vi "Get Status Info [STS].vi"(7 "Micropulse # In":i32, 8 "error in (no error)":errorcluster, 10 "Request System Status":T1 caption="[STS]") -> (0 "error out":errorcluster, 5 "Micropulse # Out":i32)   [LabVIEW 2026, in "MicroPulse_Driver.lvlib"]
doc: "Request Parameters.\n\nFormat: STS <mode>\n\nDescription:\nFor backward compatibility STS -1 can be used to find out the information contained in a RST message without resetting the MicroPulse. Other modes can be used to request various parameters from the MicroPulse.\n\nParameters:\n<mode> : \n= 0 ¨ axis locations\n= 1 ¨ MPE settings\n= 2 ¨ BKL settings\n= 5 ¨ SPA settings\n= 6 ¨ Read status of input and output lines\n= 7 ¨ Time in seconds since last power-on, RST and SRST\n= 8 ¨ System information (see section 4.5)\n= 20 ¨ System temperature readings\n= 21 ¨ Output system log (see section 4.5)\n= 22 ¨ Erase system log (see section 4.5)\n= -1 ¨ RST message\n= -2 ¨ Copy of primary system RST message when in primary/secondary mode\n= -3 ¨ Copy of secondary system RST message when in primary/secondary mode\n\nReply from MicroPulse:\nModes 0 . 5 :\n(hex) 15 Fn a a a b b b c c c d d d 0 0 0 0\nn = <mode>\naaa = 24-bit data for axis 1 (least significant byte first)\nbbb = 24-bit data for axis 2\nccc = 24-bit data for axis 3\nddd = 24-bit data for axis 4\n\nMode 5 :\n(0x15) (0xf6) (input line 15...8 level) (input line 7...0 level)\n (output line 15...8 level) (output line 7...0 level)\n (0) (0) (0) (0) (0) (0) (0) (0) (0) (0) (0) (0)\n\nMode 7 :\n(0x15) (0xf7) (0) (0)\n (4 bytes, LSByte first, of uptime in seconds)\n (4 bytes, LSByte first, since RST in seconds)\n (4 bytes, LSByte first, since SRST in seconds )\n (0) (0)\n\nMode 20 :\n(0x15) (0xf4) (TEMP in Deg C of system) (0)\n (TEMP in Deg C of processor) (0)\n (TEMP in Deg C of any secondary system) (0)\n (TEMP in Deg C of any secondary processor) (0)\n (0) (0) (0) (0) (0) (0) (0) (0)\n\nMode -1/-2/-3 :\nAs per RST message"
uses:
  MicroPulse_Driver.lvlib
  Datatypes/MP - request system status.ctl
  Private/MP-Registry Action-Enum.ctl
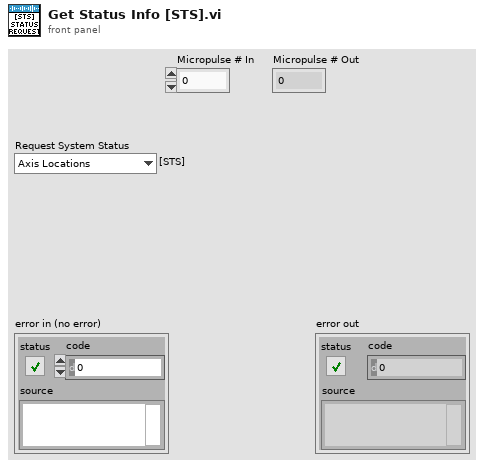
[diagram p1: front panel]
types:
  T1 = typedef "MicroPulse_Driver.lvlib/MP - request system status.ctl" = enum16{"Axis Locations", "MPE settings", "BKL settings", "SPA settings", "I/O status", "RST elapsed time", "System Status", "Temperatures", "System Log", "Erase system Log", "RST message", "Master System Msg", "Slave System Msg"}
  T2 = typedef "MicroPulse_Driver.lvlib/TCP config.ctl" = cluster{"Connection ID":refnum<k5>, "IP address":string, "host port":u16, "OC timeout":i32, "Read timeout":i32, "Write timeout":i32}
  T3 = typedef "MicroPulse_Driver.lvlib/MP-Registry Action-Enum.ctl" = enum16{"Read", "Add Test", "Add Command", "Add Gate Command", "Add Encoder Command", "Clear Command  List", "Set Registry", "Set System Details", "Set DOF", "Set Velocity", "Disable Asynch Reads", "Enable Asynch Reads", "Add Connection", "Disconnect", "Shutdown"}
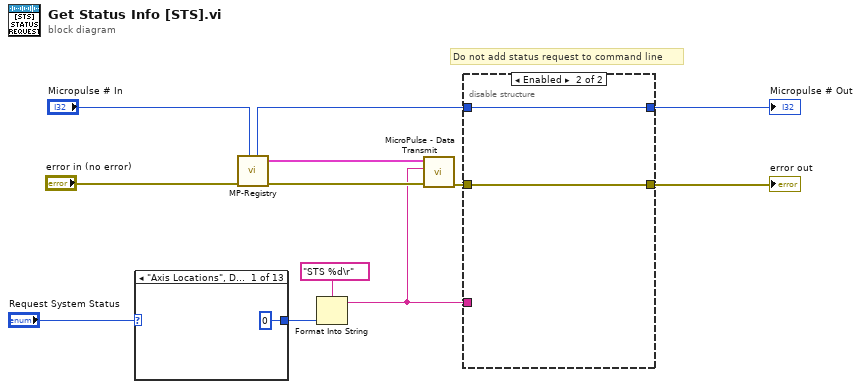
[diagram p0: block diagram]
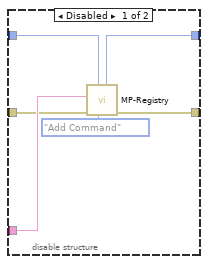
[diagram p2: hidden frame]
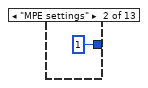
[diagram p3: hidden frame]
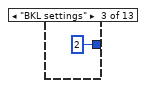
[diagram p4: hidden frame]
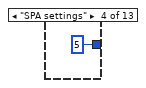
[diagram p5: hidden frame]
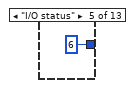
[diagram p6: hidden frame]
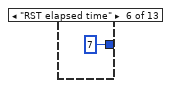
[diagram p7: hidden frame]
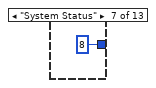
[diagram p8: hidden frame]
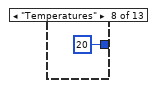
[diagram p9: hidden frame]
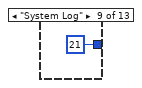
[diagram p10: hidden frame]
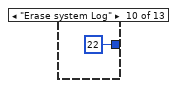
[diagram p11: hidden frame]
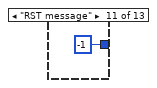
[diagram p12: hidden frame]
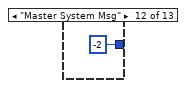
[diagram p13: hidden frame]
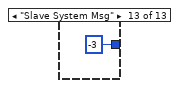
[diagram p14: hidden frame]
diagram:
  # "Do not add status request to command line"
  n1 = case shown="\"Axis Locations\", Default" "Request System Status" {
    tunnel: [0 1 2 5 6 7 8 20 21 22 -1 -2 -3] -> w1
    frame "Axis Locations", Default {
    }
    frame "MPE settings" {
    }
    frame "BKL settings" {
    }
    frame "SPA settings" {
    }
    frame "I/O status" {
    }
    frame "RST elapsed time" {
    }
    frame "System Status" {
    }
    frame "Temperatures" {
    }
    frame "System Log" {
    }
    frame "Erase system Log" {
    }
    frame "RST message" {
    }
    frame "Master System Msg" {
    }
    frame "Slave System Msg" {
    }
  }
  n2 = call "MP-Registry.vi"("Micropulse # In"="Micropulse # In", "error in (no error)"="error in (no error)") -> ("error out"=w10:errorcluster, "TCP config"=w9:T2, "Micropulse # Out"=w5:i32)  [unwired: 6 in, 1 out]
  n3 = Format Into String(format string="STS %d\r", w1) -> (resulting string=w8:string)  [unwired: 2 in, 1 out]
  n4 = call "MicroPulse - Data Transmit.vi"("error in (no error)"=w10, "data"=w8, "TCP config"=w9) -> ("error out"=w7:errorcluster)  [unwired: 6 in, 2 out]
  n5 = disable-structure shown="Enabled" {
    disable-tunnel: w8 -> [w31 _]
    disable-tunnel: w7 -> [w29 w33]
    disable-tunnel: [w28 w33] -> w6
    disable-tunnel: w5 -> [w27 w32]
    disable-tunnel: [w26 w32] -> w3
    frame Disabled {
      n6 = call "MP-Registry.vi"("Action"=MP-Registry_Action-Enum."Add Command", "Micropulse # In"=w27, "error in (no error)"=w29, "Data in"=w31) -> ("error out"=w28:errorcluster, "Micropulse # Out"=w26:i32)  [unwired: 4 in, 2 out]
    }
    frame Enabled {
    }
  }
  "error out" <- w6
  "Micropulse # Out" <- w3
